vi "Example Analog Read.vi"(8 "Index":i32, 11 "Array":dbl[](array[numeric])) -> (3 "Force (N)":dbl)   [LabVIEW 2018]
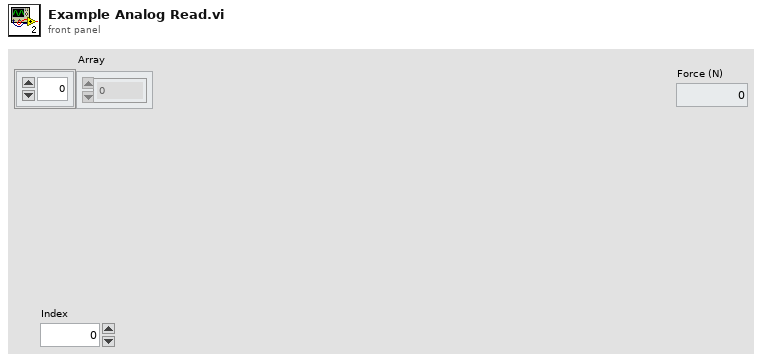
[diagram p1: front panel]
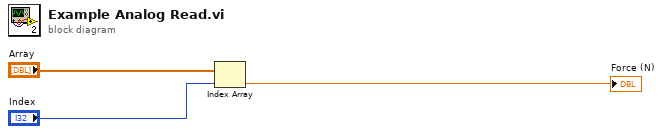
[diagram p0: block diagram]
diagram:
  n1 = Index Array "Index Array"(array="Array", index="Index") -> (element=→"Force (N)":dbl)
